vi "global autotest.vi"() -> ()   [LabVIEW 2017, in "NI_AdvCtrl_continuous linear.lvlib"]
doc: "LabVIEW no longer supports this VI. You can obtain similar functionality by installing the LabVIEW Simulation Module."
uses:
  <vilib>/addons/control/advanced/NI_AdvCtrl_continuous linear.lvlib
panel:
  in  "error":i32
  in  "auto test":bool
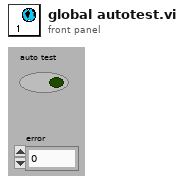
[diagram p1: front panel]
diagram:
